vi "_001.vi"() -> ()   [LabVIEW 2024]
panel:
  in  "x":dbl
  in  "y":dbl
  out "x/y":dbl
  in  "x":dbl
  in  "y":dbl
  out "x*y":dbl
  in  "x":dbl
  in  "y":dbl
  out "x-y":dbl
  out "x+y":dbl
  in  "y":dbl
  in  "x":dbl
  # "Addition :"
  # "Subtraction :"
  # "Multiplication :"
  # "Division :"
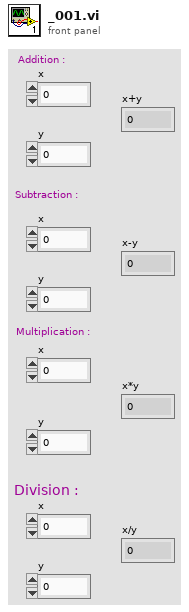
[diagram p1: front panel]
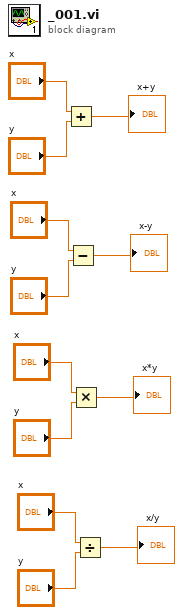
[diagram p0: block diagram]
diagram:
  n1 = Add(x="x", y="y") -> (x+y=→"x+y":dbl)
  n2 = Subtract(x="x", y="y") -> (x-y=→"x-y":dbl)
  n3 = Multiply(x="x", y="y") -> (x*y=→"x*y":dbl)
  n4 = Divide(x="x", y="y") -> (x/y=→"x/y":dbl)
